vi "initTPDO.vi"(8 "error in (no error)":errorcluster, 9 "PDO channel":u8(ring) items=["PDO 1", "PDO 2", "PDO 3", "PDO 4"], 10 "interface object in":refnum<k20>, 11 "Orion_BMS in":refnum<class "Orion_BMS.lvclass">) -> (0 "error out":errorcluster, 1 "interface object out":refnum<k20>, 2 "TPDO object out":refnum<k20>, 3 "Orion_BMS out":refnum<class "Orion_BMS.lvclass">)   [LabVIEW 2018, in "Orion_BMS.lvclass"]
uses:
  Orion_BMS.lvclass
  Orion_BMS.lvclass/Orion_BMS.ctl
  <vilib>/CANopenLib/CANOPEN.llb/CANopen TPDO Create.vi
  <vilib>/CANopenLib/CANOPEN.llb/CANopen TPDO Start.vi
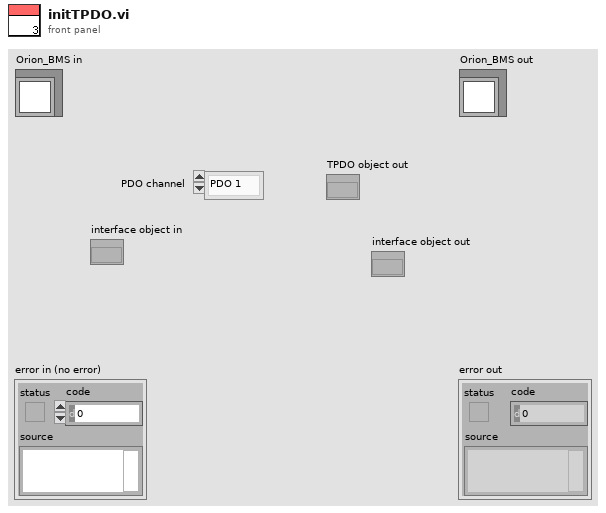
[diagram p1: front panel]
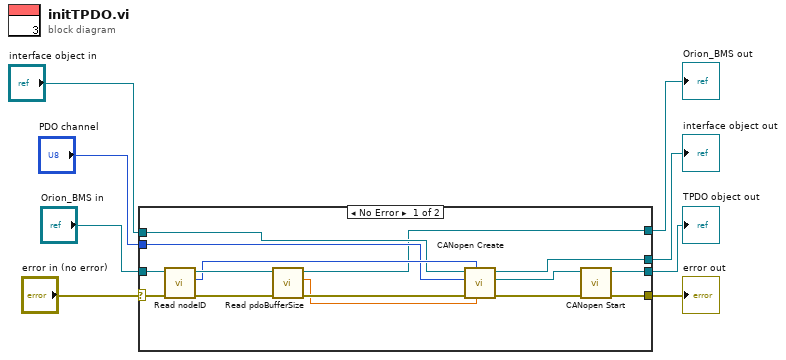
[diagram p0: block diagram]
diagram:
  n1 = case shown="No Error" "error in (no error)" {
    selector: "error in (no error)" -> [w22 w26]
    tunnel: [w10 w26] -> w2
    tunnel: [w15 w25] -> w4
    tunnel: "Orion_BMS in" -> [w23 w25]
    tunnel: "interface object in" -> [w18 w24]
    tunnel: "PDO channel" -> [w17 _]
    tunnel: [w14 w24] -> w1
    tunnel: [w12 _] -> w3
    frame No Error {
      n2 = call "Read nodeID.vi"("error in (no error)"=w22, "OrionBMS in"=w23) -> ("error out"=w21:errorcluster, "nodeID"=w19:u8, "OrionBMS out"=w20:refnum<class "Orion_BMS.lvclass">)  [unwired: 7 in]
      n3 = call "Read pdoBufferSize.vi"("error in (no error)"=w21, "OrionBMS in"=w20) -> ("error out"=w16:errorcluster, "pdoBufferSize"=w9:dbl, "OrionBMS out"=w15:refnum<class "Orion_BMS.lvclass">)  [unwired: 7 in]
      n4 = call-poly <vilib>:"CANopen Create.vi"("buffer size (0)"=w9, "node-ID"=w19, "error in (no error)"=w16, "PDO channel"=w17, "interface object in"=w18) -> ("error out"=w11:errorcluster, "TPDO object out"=w13:refnum<k20>, "interface object out"=w14:refnum<k20>)  [unwired: 4 in]
      n5 = call-poly <vilib>:"CANopen Start.vi"("error in (no error)"=w11, "TPDO object in"=w13) -> ("error out"=w10:errorcluster, "TPDO object out"=w12:refnum<k20>)  [unwired: 8 in]
    }
    frame Error {
    }
  }
  "error out" <- w2
  "Orion_BMS out" <- w4
  "TPDO object out" <- w3
  "interface object out" <- w1
